vi "lv receive.vi"(7 "flags":i32, 8 "error in":errorcluster, 11 "socket":i64) -> (0 "error out":errorcluster, 2 "data":string)   [LabVIEW 2013, in "lvnano.lvlib"]
doc: "NN_EXPORT int nn_recv (int s, void *buf, size_t len, int flags);"
uses:
  lvnano.lvlib
  get last error code.vi
  get error string from code.vi
  <vilib>/Utility/error.llb/Error Cluster From Error Code.vi
  lvnanomsg.dll
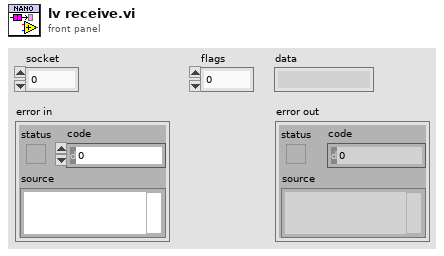
[diagram p1: front panel]
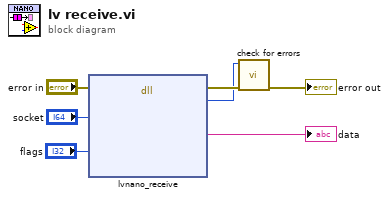
[diagram p0: block diagram]
diagram:
  n1 = dll-call lib="C:/Users/Daniel/Documents/nanomsg/lvnano/lvnanomsg.*" fn="lvnano_receive"(error in="error in", "socket"="socket", "flags"="flags") -> (error out=w4:errorcluster, "message size"=w3:i32, "data buffer"=→"data":string)  [unwired: 7 in, 1 out]
  n2 = call "check for errors.vi"("error in"=w4, "function return"=w3) -> ("error out"=→"error out":errorcluster)  [unwired: 9 in]
